vi "BMark_OpenWindow.vi"(8 "error in (no error)":errorcluster, 11 "Bookmark manager window reference":refnum<vi>) -> (0 "error out":errorcluster, 2 "bounds":T1, 3 "Bookmark manager window reference out":refnum<vi>)   [LabVIEW 2018]
uses:
  <resource>/dialog/lvconfig.llb/LV Config Read String.vi
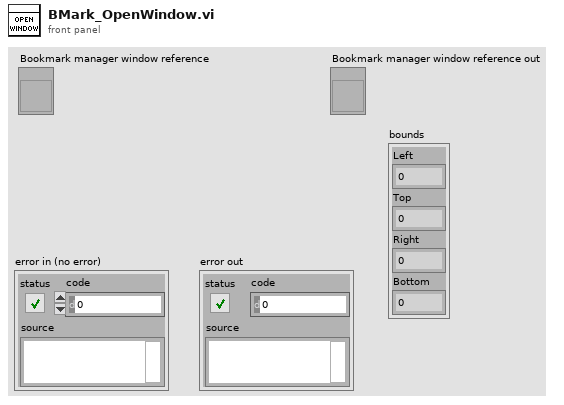
[diagram p1: front panel]
types:
  T1 = cluster{"Left":i16, "Top":i16, "Right":i16, "Bottom":i16}
  T2 = enum32{"Invalid", "Standard", "Closed", "Hidden", "Minimized", "Maximized"}
  T3 = typedef "LVAllMonitorsDisplayTypeDef.ctl" = cluster{"Bounds":cluster{"Left":i16, "Top":i16, "Right":i16, "Bottom":i16}, "Depth":i16}[]
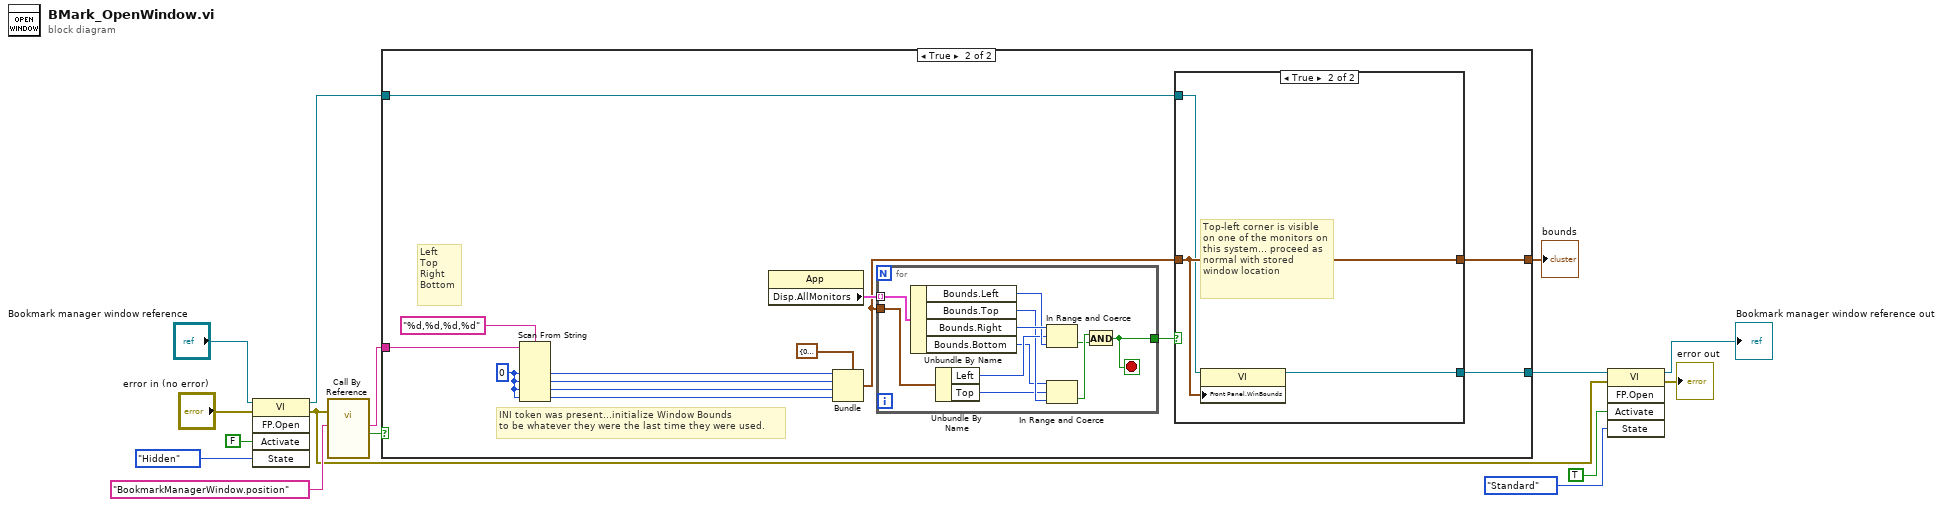
[diagram p0: block diagram]
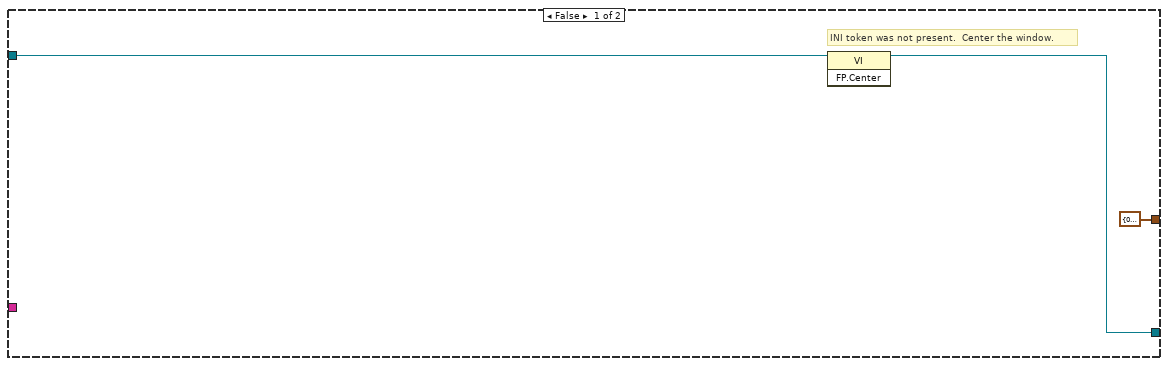
[diagram p2: hidden frame]
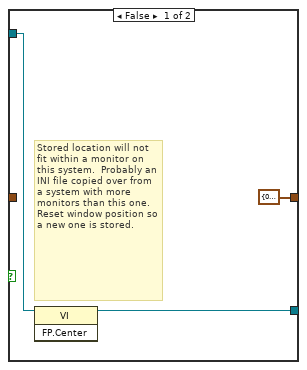
[diagram p3: hidden frame]
diagram:
  n1 = invoke class="VI" method="FP.Open"(reference="Bookmark manager window reference", error in="error in (no error)", "Activate"=FALSE ("Activate?"), "State"=T2."Hidden") -> (reference out=w6:refnum<vi>, error out=w2:errorcluster)  [unwired: 1 in, 3 out]
  n2 = call-by-ref "?"(error in=w2, "key"="BookmarkManagerWindow.position") -> ("found?"=w7:bool, "value"=w9:string)  [unwired: 5 in, 3 out]
  n3 = case shown="True" w7 {
    tunnel: [T1 {"Left"=0, "Top"=0, "Right"=0, "Bottom"=0} ("Front Panel.PanelBounds") w21] -> w1
    tunnel: w9 -> [_ w32]
    tunnel: w6 -> [w17 w20]
    tunnel: [w16 w19] -> w5
    frame False {
      # "INI token was not present.  Center the window."
      n4 = invoke class="VI" method="FP.Center"(reference=w17) -> (reference out=w16:refnum<vi>)  [unwired: 2 in, 2 out]
    }
    frame True {
      w30 = i16 0 ("default value 1")
      # "Left\nTop\nRight\nBottom"
      # "INI token was present...initialize Window Bounds\nto be whatever they were the last time they were used."
      n5 = Scan From String(format string="%d,%d,%d,%d", input string=w32, default 1=w30, default 2=w30, default 3=w30, default 4=w30) -> (output 1=w29:i16, output 2=w28:i16, output 3=w27:i16, output 4=w26:i16)  [unwired: 2 in, 3 out]
      n6 = property class="App"() -> ("Disp.AllMonitors"=w24:T3)  [unwired: 2 in, 2 out]
      n7 = Bundle(cluster=T1 {"Left"=0, "Top"=0, "Right"=0, "Bottom"=0} ("Front Panel.PanelBounds"), "Left"=w29, "Top"=w28, "Right"=w27, "Bottom"=w26) -> (w23:T1)
      n8 = for {
        tunnel: w24 -> [w49] mode=indexing
        tunnel: w23 -> [w48]
        tunnel: [w39] -> w22
        stop <- w39 stop-if-true
        n9 = Unbundle By Name(w49) -> ("Bounds.Left"=w46:i16, "Bounds.Top"=w44:i16, "Bounds.Right"=w47:i16, "Bounds.Bottom"=w43:i16)
        n10 = Unbundle By Name(w48) -> ("Left"=w45:i16, "Top"=w42:i16)
        n11 = In Range and Coerce(upper limit=w47, x=w45, lower limit=w46) -> (In Range?=w40:bool)  [unwired: 1 out]
        n12 = In Range and Coerce(upper limit=w43, x=w42, lower limit=w44) -> (In Range?=w41:bool)  [unwired: 1 out]
        n13 = And(x=w41, y=w40) -> (x .and. y?=w39:bool)
      }
      n14 = case shown="True" w22 {
        tunnel: w23 -> [_ w38]
        tunnel: [T1 {"Left"=0, "Top"=0, "Right"=0, "Bottom"=0} ("Front Panel.PanelBounds") w38] -> w21
        tunnel: w20 -> [w34 w37]
        tunnel: [w33 w36] -> w19
        frame False {
          # "Stored location will not fit within a monitor on this system.  Probably an INI file copied over from a system with more monitors than this one.  Reset window position so a new one is stored."
          n15 = invoke class="VI" method="FP.Center"(reference=w34) -> (reference out=w33:refnum<vi>)  [unwired: 2 in, 2 out]
        }
        frame True {
          # "Top-left corner is visible on one of the monitors on this system... proceed as normal with stored window location"
          n16 = property class="VI"(reference=w37, "Front Panel.WinBounds"=w38) -> (reference out=w36:refnum<vi>)  [unwired: 1 in, 1 out]
        }
      }
    }
  }
  "bounds" <- w1
  n17 = invoke class="VI" method="FP.Open"(reference=w5, error in=w2, "Activate"=TRUE ("Activate?"), "State"=T2."Standard") -> (reference out=→"Bookmark manager window reference out":refnum<vi>, error out=→"error out":errorcluster)  [unwired: 1 in, 3 out]
